vi "RESTful Check Reserved Terminal.vi"(10 "Terminal Info Summary":T1) -> (2 "reserved terminal?":bool)   [LabVIEW 2020]
uses:
  <vilib>/AppBuilder/Engine/RESTful INI Generator/RESTful VI Terminal Info Summary.ctl
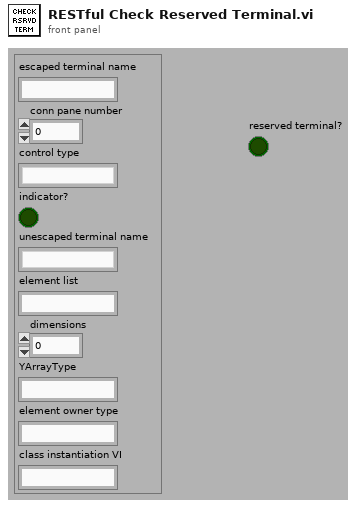
[diagram p1: front panel]
types:
  T1 = typedef "RESTful VI Terminal Info Summary.ctl" = cluster{"escaped terminal name":string, "conn pane number":i32, "control type":string, "indicator?":bool, "unescaped terminal name":string, "element list":string, "dimensions":u32, "YArrayType":string, "element owner type":string, "class instantiation VI":string}
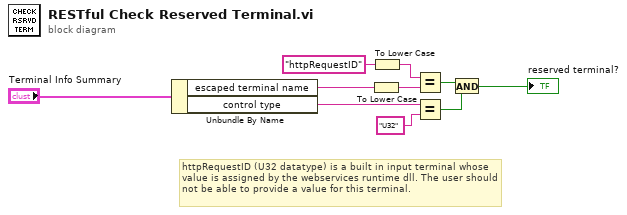
[diagram p0: block diagram]
diagram:
  # "httpRequestID (U32 datatype) is a built in input terminal whose value is assigned by the webservices runtime dll. The user should not be able to provide a value for this terminal."
  n1 = Unbundle By Name("Terminal Info Summary") -> ("escaped terminal name"=w2:string, "control type"=w9:string)
  n2 = To Lower Case(string=w2) -> (all lower case string=w5:string)
  n3 = To Lower Case(string="httpRequestID" ("x")) -> (all lower case string=w6:string)
  n4 = Equal?(x=w6, y=w5) -> (x = y?=w4:bool)
  n5 = Equal?(x=w9, y="U32") -> (x = y?=w3:bool)
  n6 = And(x=w4, y=w3) -> (x .and. y?=→"reserved terminal?":bool)
